vi "2D Brown motion of a particle.vi"() -> ()   [LabVIEW 2016]
uses:
  <vilib>/Analysis/NI_AALBase.lvlib
panel:
  out "3D Brown mozgás elmozdulásának\n hisztogramja":T1(graph)
  out "futtatások száma":i32
  out "a részecske összes megtett útja":dbl
  out "3D Brown mozgás XY vetülete":cluster{dbl[], dbl[]}(graph)
  out "a részecske által megtett\n út ciklusonként":dbl
  in  "lépések száma":i32
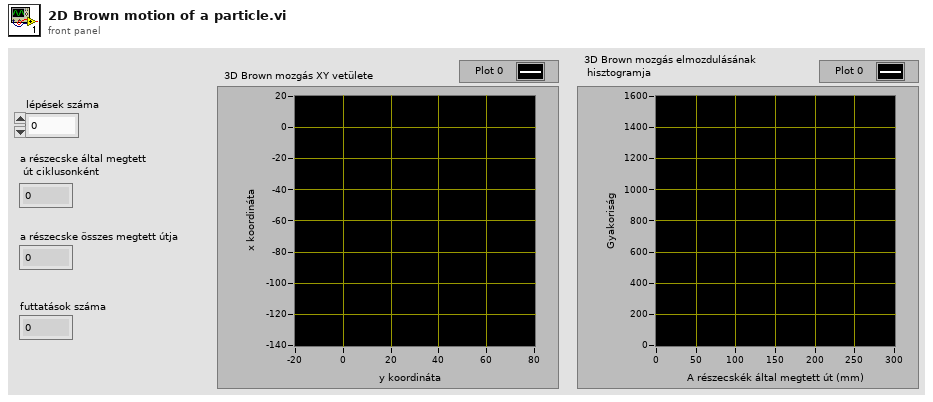
[diagram p1: front panel]
types:
  T1 = cluster{"X Values":dbl[], "Histogram: h(x)":i32[]}
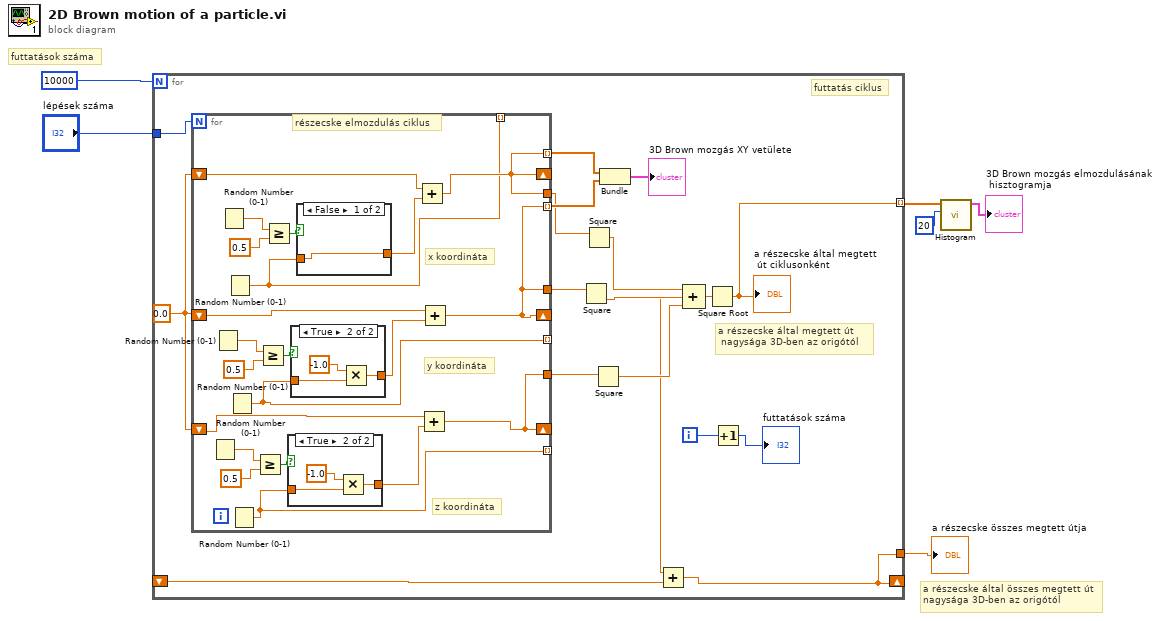
[diagram p0: block diagram]
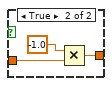
[diagram p2: hidden frame]
diagram:
  # "a részecske által összes megtett út\nnagysága 3D-ben az origótól"
  # "futtatások száma"
  n1 = for {
    N: 10000 -> [_]
    shift-right: [w16] -> _
    shift-left: _ -> [w17]
    tunnel: [w16] -> w5
    tunnel: "lépések száma" -> [w11]
    tunnel: [w10] -> w2 mode=indexing
    i -> [w15]
    w23 = 0.0
    # "a részecske által megtett út\n nagysága 3D-ben az origótól"
    # "futtatás ciklus"
    n2 = for {
      N: w11 -> [_]
      shift-right: [w31] -> _
      shift-left: w23 -> [w44]
      shift-right: [w24] -> _
      shift-left: w23 -> [w35]
      shift-right: [w42] -> _
      shift-left: w23 -> [w43]
      tunnel: [w31] -> w9
      tunnel: [w42] -> w7
      tunnel: [w31] -> w13 mode=indexing
      tunnel: [w24] -> w12 mode=indexing
      tunnel: [w24] -> w8
      tunnel: [w27] -> _ mode=indexing
      tunnel: [w26] -> _ mode=indexing
      tunnel: [w25] -> _ mode=indexing
      # "részecske elmozdulás ciklus"
      # "z koordináta"
      # "y koordináta"
      # "x koordináta"
      n3 = Random Number (0-1)() -> (number: 0 to 1=w40:dbl)
      n4 = Random Number (0-1)() -> (number: 0 to 1=w37:dbl)
      n5 = Random Number (0-1)() -> (number: 0 to 1=w33:dbl)
      n6 = Random Number (0-1)() -> (number: 0 to 1=w27:dbl)
      n7 = Random Number (0-1)() -> (number: 0 to 1=w26:dbl)
      n8 = Random Number (0-1)() -> (number: 0 to 1=w25:dbl)
      n9 = Greater Or Equal?(x=w40, y=0.5) -> (x >= y?=w41:bool)
      n10 = Greater Or Equal?(x=w37, y=0.5) -> (x >= y?=w38:bool)
      n11 = Greater Or Equal?(x=w33, y=0.5) -> (x >= y?=w34:bool)
      n12 = case shown="True" w41 {
        tunnel: w25 -> [w53 w55]
        tunnel: [w53 w54] -> w28
        frame False {
        }
        frame True {
          n13 = Multiply(x=-1.0 ("y"), y=w55) -> (x*y=w54:dbl)
        }
      }
      n14 = case shown="True" w38 {
        tunnel: w26 -> [w49 w51]
        tunnel: [w49 w50] -> w29
        frame False {
        }
        frame True {
          n15 = Multiply(x=-1.0 ("y"), y=w51) -> (x*y=w50:dbl)
        }
      }
      n16 = case shown="False" w34 {
        tunnel: w27 -> [w45 w47]
        tunnel: [w45 w46] -> w30
        frame False {
        }
        frame True {
          n17 = Multiply(x=-1.0 ("y"), y=w47) -> (x*y=w46:dbl)
        }
      }
      n18 = Add(x=w44, y=w30) -> (x+y=w31:dbl)
      n19 = Add(x=w43, y=w28) -> (x+y=w42:dbl)
      n20 = Add(x=w35, y=w29) -> (x+y=w24:dbl)
    }
    n21 = Square(x=w8) -> (x^2=w21:dbl)
    n22 = Square(x=w9) -> (x^2=w22:dbl)
    n23 = Square(x=w7) -> (x^2=w20:dbl)
    n24 = Bundle(w13, w12) -> (→"3D Brown mozgás XY vetülete":cluster{dbl[], dbl[]})  [unwired: 1 in]
    n25 = Compound Arithmetic op=ADD(w22, w21, w20) -> (w19:dbl)
    n26 = Square Root(x=w19) -> (sqrt(x)=w10:dbl)
    "a részecske által megtett\n út ciklusonként" <- w10
    n27 = Add(x=w10, y=w17) -> (x+y=w16:dbl)
    n28 = Increment(x=w15) -> (x+1=→"futtatások száma":i32)
  }
  "a részecske összes megtett útja" <- w5
  n29 = call <vilib>:"Histogram.vi"("intervals"=20, "X"=w2) -> ("Histogram Graph"=→"3D Brown mozgás elmozdulásának\n hisztogramja":T1)  [unwired: 6 in, 3 out]
